vi "FileCreatorMain.vi"() -> ()   [LabVIEW 2017]
uses:
  AutoFileDataType.ctl
panel:
  in  "Flip This Auto":bool
  in  "Auto":T1
  in  "Path File Name":string[](array[string])
  out "standard output":string
  out "standard error":string="NI Linux Real-Time (run mode)\n\nLog in with your NI-Auth credentials.\n\n"
  in  "ExportAllToRobot":bool
  in  "SaveToLocal":bool
  in  "LoadFromLocal":bool
  in  "ExportToRobot":bool
  in  "LoadAllFromRobot":bool
  in  "LocalFiles":i32(listbox)=2
  in  "LocalFileNames":string[](array[string])=["1A.txt", "1B.txt", "1C.txt", "1D.txt", "2A.txt", "2B.txt", "2C.txt", "2D.txt", "3A.txt", "3B.txt", "3C.txt", "3D.txt", "4A.txt", "4B.txt", "4C.txt", "4D.txt"]
  # "Drive:\nWait or\nStart"
  # "Elevator:\nWait or\nStart"
  # "Intake:\nWait or\nStart"
  # "Distance \nfor\nElevator"
  # "Degrees \nto turn"
  # "Elevator\nCommand"
  # "Time for \nintake"
  # "Drive\ncommand"
  # "Time\nfor elevator"
  # "Elevator\n Speed"
  # "Intake \nCommand"
  # "Path File Path"
  # "Speed"
  # "Distance(in)"
  # "Intake Speed"
  # "Drive commands:\n1. For time\n2. For distance\n3. Turn for angle\n4. Stop\n5. Drive Path\n6. Turn To Angle"
  # "Elevator Commands:\n1. For time\n2. To distance\n3. Stop\n4. Pause for time, then distance"
  # "Intake Commands:\n1. For time\n2. Until cube\n3. Stop"
  # "Wait: 0\nStart: 1"
  # "Responses of CMDs run"
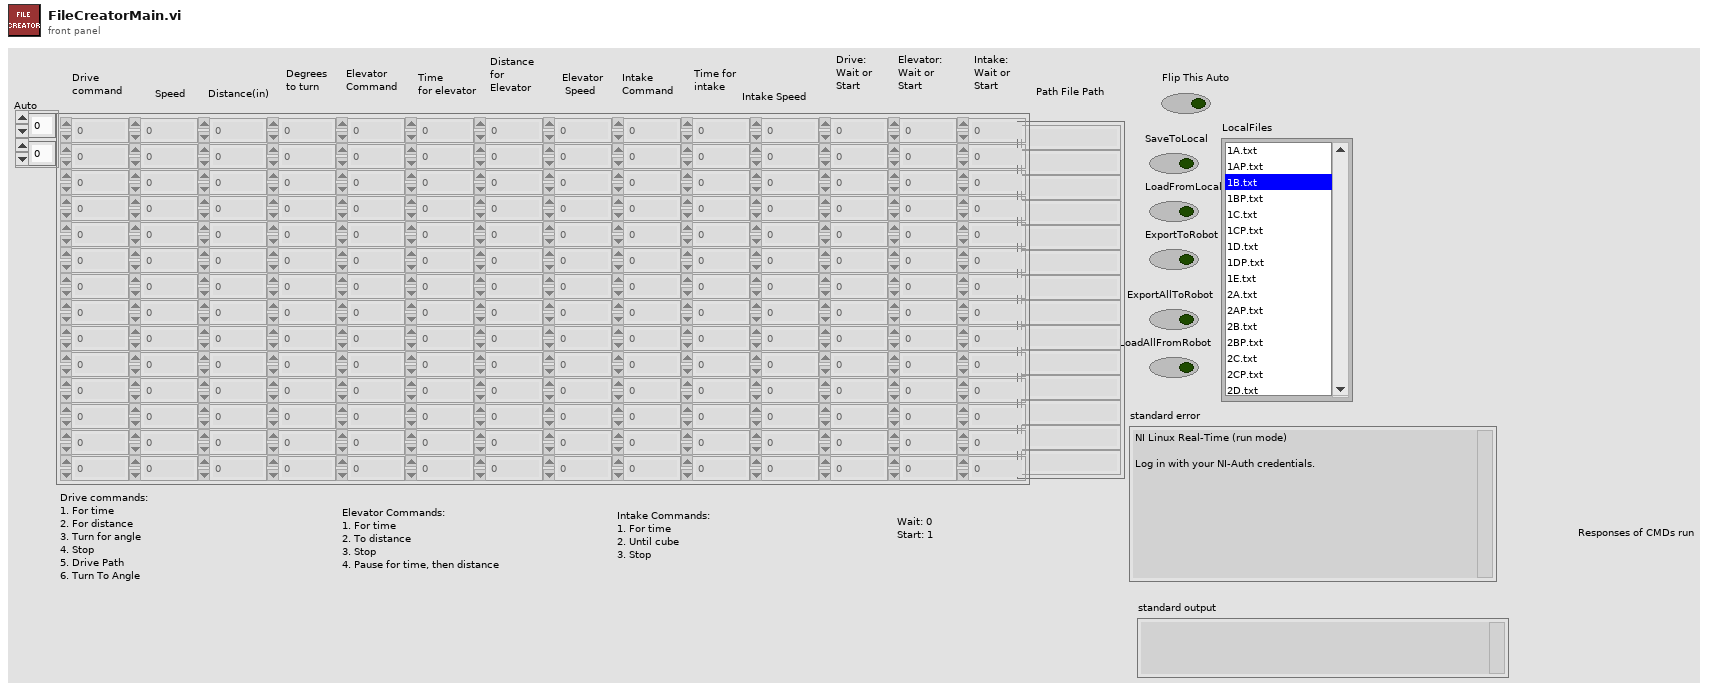
[diagram p1: front panel]
types:
  T1 = typedef "AutoFileDataType.ctl" = dbl[][]
  T2 = enum16{"open", "replace", "create", "open or create", "replace or create", "replace or create with confirmation"}
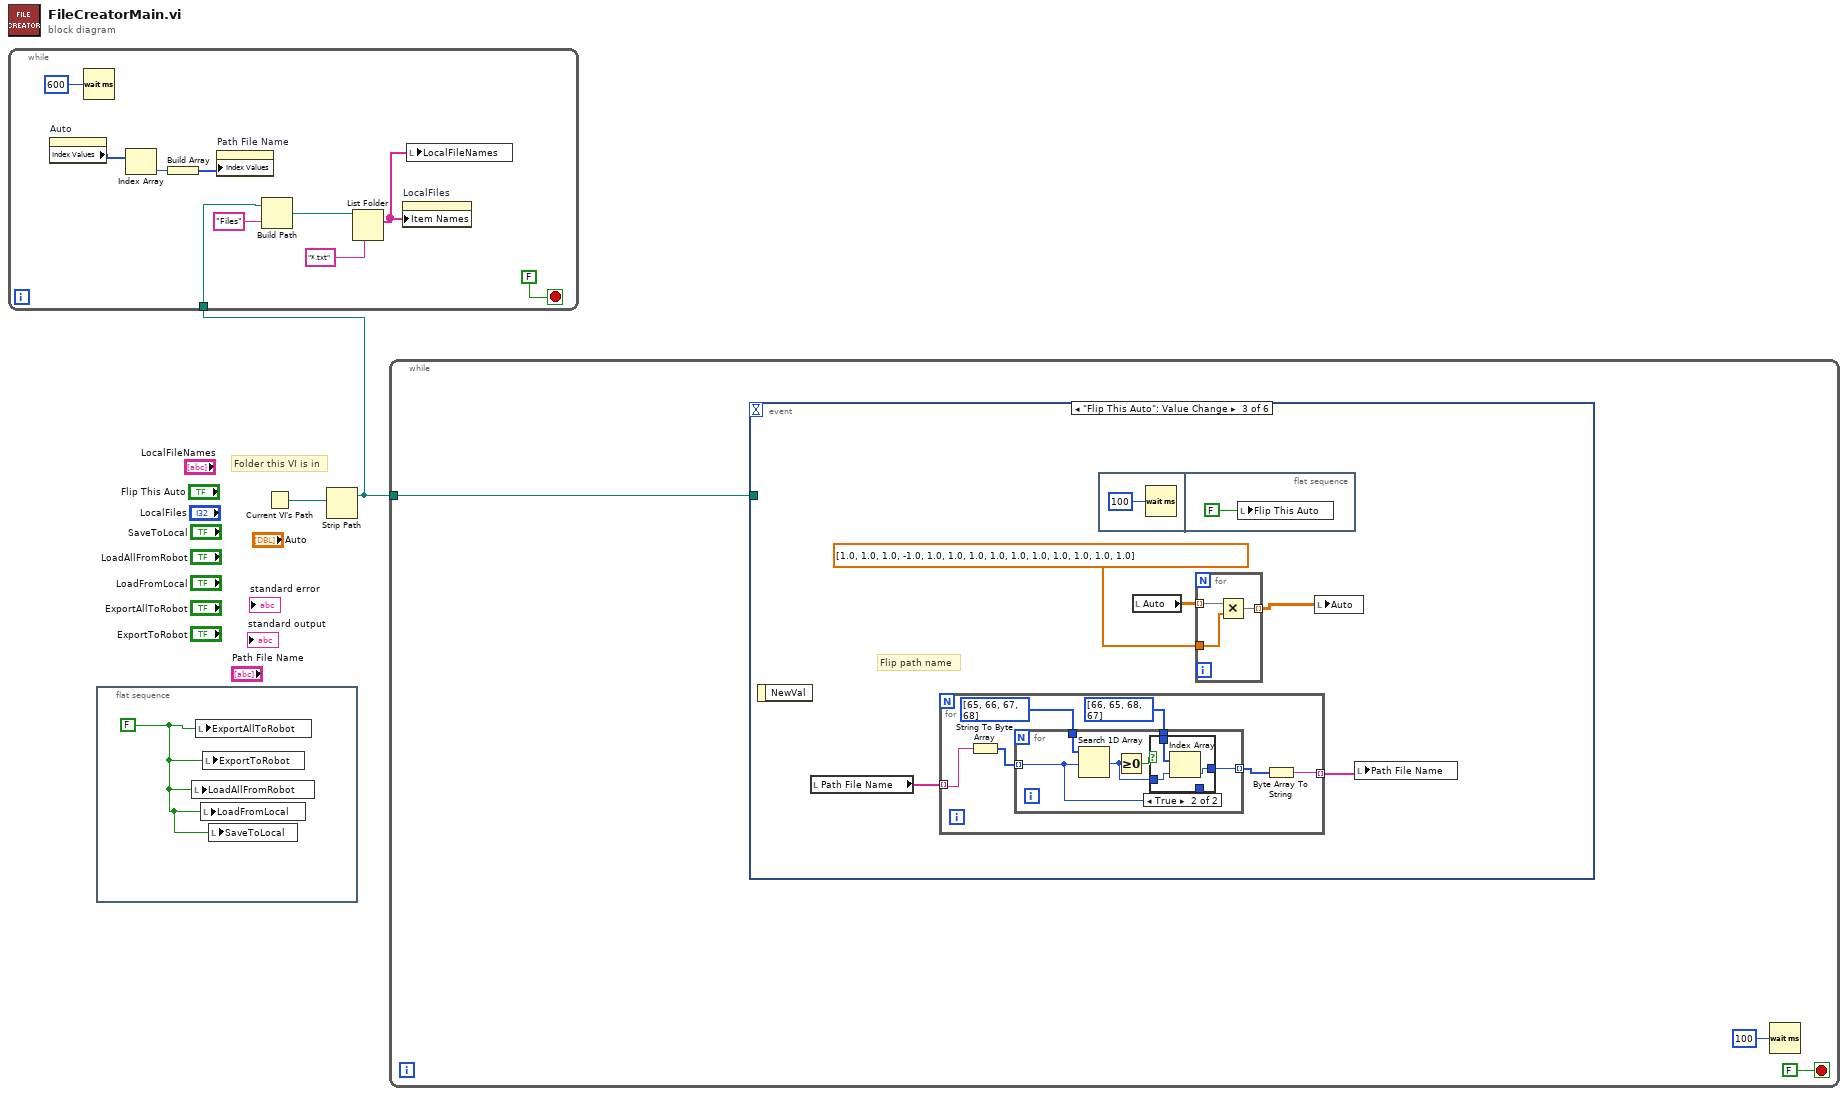
[diagram p0: block diagram]
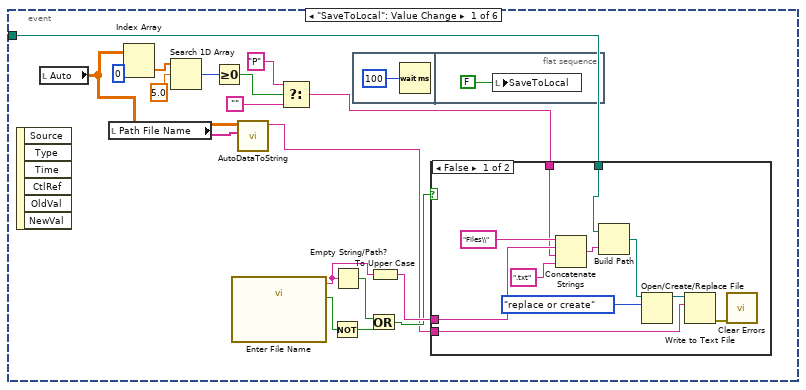
[diagram p2: hidden frame]
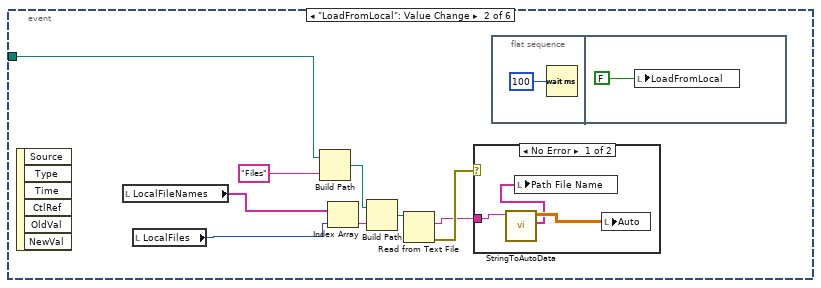
[diagram p4: hidden frame]
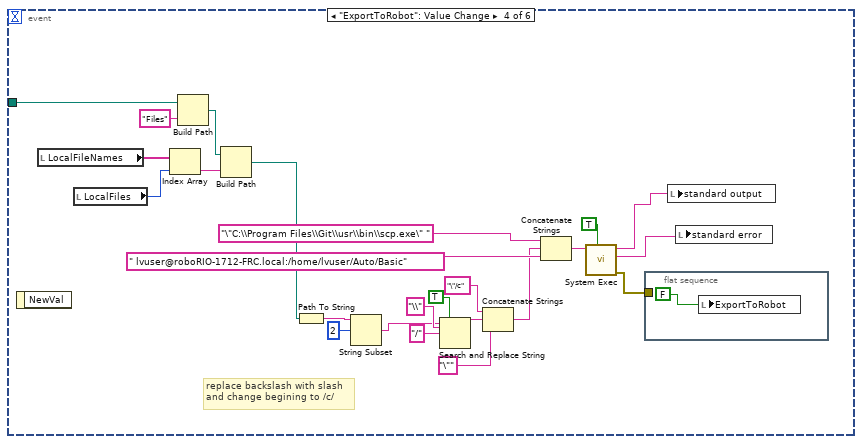
[diagram p7: hidden frame]
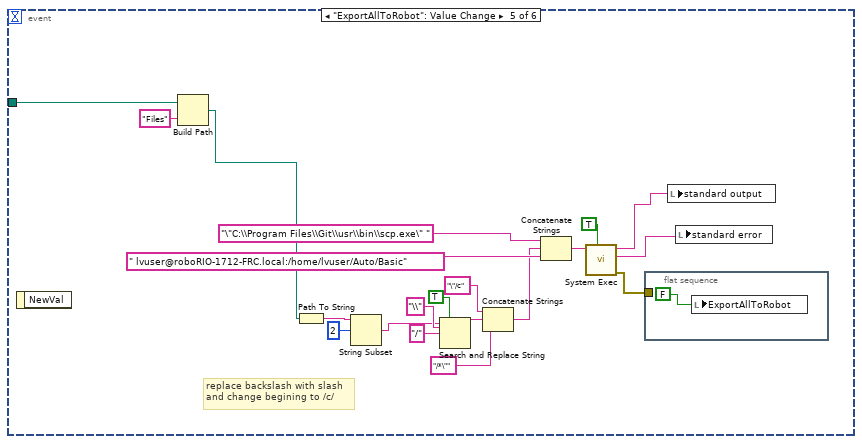
[diagram p8: hidden frame]
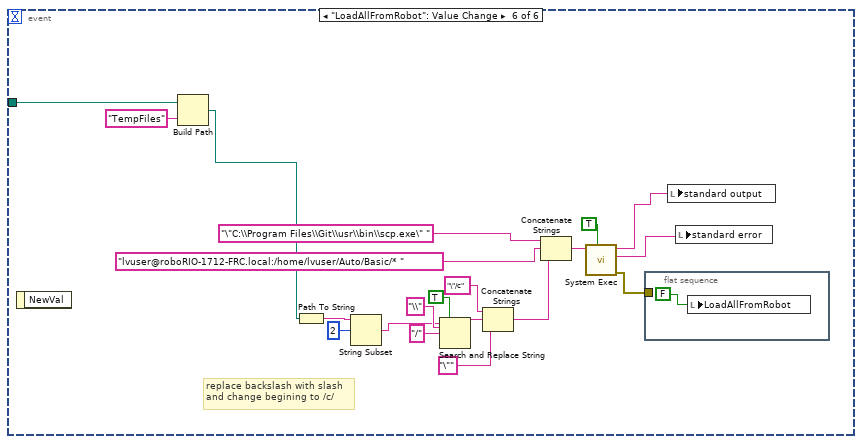
[diagram p9: hidden frame]
diagram:
  # "Folder this VI is in"
  n1 = flat-sequence {
    frame #0 {
      w3 = FALSE ("ExportToRobot")
      n2 = local write "LoadAllFromRobot"(w3) -> ()
      n3 = local write "ExportAllToRobot"(w3) -> ()
      n4 = local write "LoadFromLocal"(w3) -> ()
      n5 = local write "ExportToRobot"(w3) -> ()
      n6 = local write "SaveToLocal"(w3) -> ()
    }
  }
  n7 = Current VI's Path() -> (path=w2:path)
  n8 = Strip Path(path=w2) -> (stripped path=w1:path)  [unwired: 1 out]
  n9 = while {
    tunnel: w1 -> [w9]
    stop <- FALSE stop-if-true
    n10 = property on="Auto" class="Arr (strict)"() -> ("Index Values"=w6:u32[])  [unwired: 2 in, 2 out]
    n11 = Wait (ms)(milliseconds to wait=u32 600) -> ()  [unwired: 1 out]
    n12 = Index Array(array=w6) -> (element=w5:u32)  [unwired: 1 in]
    n13 = Build Array(w5) -> (w4:u32[])
    n14 = property on="Path File Name" class="Arr (strict)"("Index Values"=w4) -> ()  [unwired: 2 in, 2 out]
    n15 = Build Path(base path=w9, name or relative path="Files") -> (appended path=w11:path)
    n16 = List Folder(path=w11, pattern="*.txt") -> (filenames=w7:string[])  [unwired: 2 in, 3 out]
    n17 = property on="LocalFiles" class="LstBox (strict)"("Item Names"=w7) -> ()  [unwired: 2 in, 2 out]
    n18 = local write "LocalFileNames"(w7) -> ()
  }
  n19 = while {
    tunnel: w1 -> [w15]
    stop <- FALSE stop-if-true
    n20 = event shown="[2] \"Flip This Auto\": Value Change" {
      selector: _ -> [_ _ _ _ _ _]
      dyn-events: _ -> [_ _ _ _ _ _]
      timeout: _ -> [_ _ _ _ _ _]
      tunnel: w15 -> [w28 w52 _ w106 w131 w152]
      event "SaveToLocal": Value Change {
        n21 = event-data() -> ()  [unwired: 1 in, 6 out]
        n22 = local read "Auto"() -> (w25:T1)
        n23 = local read "Path File Name"() -> (w26:string[])
        n24 = Index Array(array=w25, index (col)=0 ("disabled index (col)")) -> (element=w24:dbl[])  [unwired: 1 in]
        n25 = Search 1D Array(1D array=w24, element=5.0) -> (index of element=w22:i32)  [unwired: 1 in]
        n26 = Greater Or Equal To 0?(x=w22) -> (x >= 0?=w21:bool)
        n27 = call "Enter File Name"() -> ("File Name"=w31:string, "Enter"=w33:bool)  [unwired: 17 in, 1 out]
        n28 = call "AutoDataToString.vi"("File Path Name"=w26, "Auto"=w25) -> ("String"=w27:string)  [unwired: 9 in]
        n29 = Select(t="P", s=w21, f="") -> (s? t:f=w18:string)
        n30 = Not(x=w33) -> (.not. x?=w32:bool)
        n31 = Empty String/Path?(string/path=w31) -> (empty?=w34:bool)
        n32 = flat-sequence {
          frame #0 {
            n33 = Wait (ms)(milliseconds to wait=u32 100) -> ()  [unwired: 1 out]
          }
          frame #1 {
            n34 = local write "SaveToLocal"(FALSE ("SaveToLocal")) -> ()
          }
        }
        n35 = Or(x=w34, y=w32) -> (x .or. y?=w29:bool)
        n36 = To Upper Case(1:w31) -> (0:w30:string)
        n37 = case shown="False" w29 {
          tunnel: w30 -> [w44 _]
          tunnel: w27 -> [w43 _]
          tunnel: w28 -> [w39 _]
          tunnel: w18 -> [w37 _]
          frame False {
            n38 = Concatenate Strings("Files\\" ("name or relative path"), w44, w37, ".txt" ("string")) -> (w47:string)
            n39 = Build Path(base path=w39, name or relative path=w47) -> (appended path=w42:path)
            n40 = Open/Create/Replace File(file path (use dialog)=w42, operation (0:open)=T2."replace or create") -> (refnum out=w41:refnum<file>)  [unwired: 4 in, 2 out]
            n41 = Write to Text File(file (use dialog)=w41, text=w43) -> (error out=w45:errorcluster)  [unwired: 2 in, 2 out]
            n42 = call <vilib>:"Clear Errors.vi"("error in (no error)"=w45) -> ()  [unwired: 5 in, 2 out]
          }
          frame True {
          }
        }
      }
      event "LoadFromLocal": Value Change {
        n43 = event-data() -> ()  [unwired: 1 in, 6 out]
        n44 = local read "LocalFileNames"() -> (w51:string[])
        n45 = local read "LocalFiles"() -> (w50:i32)
        n46 = Build Path(base path=w52, name or relative path="Files") -> (appended path=w55:path)
        n47 = Index Array(array=w51, index=w50) -> (element=w54:string)
        n48 = Build Path(base path=w55, name or relative path=w54) -> (appended path=w53:path)
        n49 = Read from Text File(file (use dialog)=w53) -> (text=w48:string, error out=w49:errorcluster)  [unwired: 3 in, 2 out]
        n50 = case shown="No Error" w49 {
          tunnel: w48 -> [w61 _]
          frame No Error {
            n51 = call "StringToAutoData.vi"("String"=w61) -> ("Path File Names"=w59:string[], "Auto"=w60:T1)  [unwired: 9 in]
            n52 = local write "Path File Name"(w59) -> ()
            n53 = local write "Auto"(w60) -> ()
          }
          frame Error {
          }
        }
        n54 = flat-sequence {
          frame #0 {
            n55 = Wait (ms)(milliseconds to wait=u32 100) -> ()  [unwired: 1 out]
          }
          frame #1 {
            n56 = local write "LoadFromLocal"(FALSE ("SaveToLocal")) -> ()
          }
        }
      }
      event "Flip This Auto": Value Change {
        # "Flip path name"
        n57 = event-data() -> ()  [unwired: 1 in, 1 out]
        n58 = local read "Path File Name"() -> (w63:string[])
        n59 = for {
          tunnel: w63 -> [w70] mode=indexing
          tunnel: [w68] -> w62 mode=indexing
          n60 = String To Byte Array(string=w70) -> (unsigned byte array=w72:u8[])
          n61 = for {
            tunnel: w72 -> [w75] mode=indexing
            tunnel: u8[] [65, 66, 67, 68] ("1D array") -> [w78]
            tunnel: [w76] -> w69 mode=indexing
            tunnel: u8[] [66, 65, 68, 67] ("1D array") -> [w73]
            n62 = Search 1D Array(1D array=w78, element=w75) -> (index of element=w74:i32)  [unwired: 1 in]
            n63 = Greater Or Equal To 0?(x=w74) -> (x >= 0?=w77:bool)
            n64 = case shown="True" w77 {
              tunnel: [w79 w82] -> w76
              tunnel: w75 -> [w79 _]
              tunnel: w74 -> [_ w81]
              tunnel: w73 -> [_ w80]
              frame False {
              }
              frame True {
                n65 = Index Array(array=w80, index=w81) -> (element=w82:u8)
              }
            }
          }
          n66 = Byte Array To String(unsigned byte array=w69) -> (string=w68:string)
        }
        n67 = flat-sequence {
          frame #0 {
            n68 = Wait (ms)(milliseconds to wait=u32 100) -> ()  [unwired: 1 out]
          }
          frame #1 {
            n69 = local write "Flip This Auto"(FALSE ("Flip This Auto")) -> ()
          }
        }
        n70 = local read "Auto"() -> (w65:T1)
        n71 = for {
          tunnel: dbl[] [1.0, 1.0, 1.0, -1.0, 1.0, 1.0, 1.0, 1.0, 1.0, 1.0, 1.0, 1.0, 1.0, 1.0] -> [w87]
          tunnel: w65 -> [w86] mode=indexing
          tunnel: [w85] -> w64 mode=indexing
          n72 = Multiply(x=w86, y=w87) -> (x*y=w85:dbl[])
        }
        n73 = local write "Auto"(w64) -> ()
        n74 = local write "Path File Name"(w62) -> ()
      }
      event "ExportToRobot": Value Change {
        # "replace backslash with slash\nand change begining to /c/"
        n75 = event-data() -> ()  [unwired: 1 in, 1 out]
        n76 = local read "LocalFileNames"() -> (w109:string[])
        n77 = local read "LocalFiles"() -> (w108:i32)
        n78 = Index Array(array=w109, index=w108) -> (element=w110:string)
        n79 = Build Path(base path=w106, name or relative path="Files") -> (appended path=w111:path)
        n80 = Build Path(base path=w111, name or relative path=w110) -> (appended path=w90:path)
        n81 = Path To String(path=w90) -> (string=w98:string)
        n82 = String Subset(string=w98, offset (0)=2) -> (substring=w96:string)  [unwired: 1 in]
        n83 = Search and Replace String(replace all?=TRUE ("replace all? (F)"), input string=w96, search string="\\", replace string="/" ("replace string (\"\")")) -> (result string=w95:string)  [unwired: 4 in, 3 out]
        n84 = Concatenate Strings("\"/c" ("string"), w95, "\"" ("string")) -> (w93:string)
        n85 = Concatenate Strings("\"C:\\Program Files\\Git\\usr\\bin\\scp.exe\" " ("command line"), w93, " lvuser@roboRIO-1712-FRC.local:/home/lvuser/Auto/Basic" ("string")) -> (w102:string)
        n86 = call <vilib>:"System Exec.vi"("wait until completion? (T)"=TRUE, "command line"=w102) -> ("error out"=w91:errorcluster, "standard error"=w89:string, "standard output"=w88:string)  [unwired: 6 in, 1 out]
        n87 = flat-sequence {
          tunnel: w91 -> [_]
          frame #0 {
            n88 = local write "ExportToRobot"(FALSE ("Export To File")) -> ()
          }
        }
        n89 = local write "standard output"(w88) -> ()
        n90 = local write "standard error"(w89) -> ()
      }
      event "ExportAllToRobot": Value Change {
        # "replace backslash with slash\nand change begining to /c/"
        n91 = event-data() -> ()  [unwired: 1 in, 1 out]
        n92 = Build Path(base path=w131, name or relative path="Files") -> (appended path=w113:path)
        n93 = Path To String(path=w113) -> (string=w123:string)
        n94 = String Subset(string=w123, offset (0)=2) -> (substring=w121:string)  [unwired: 1 in]
        n95 = Search and Replace String(replace all?=TRUE ("replace all? (F)"), input string=w121, search string="\\", replace string="/" ("replace string (\"\")")) -> (result string=w120:string)  [unwired: 4 in, 3 out]
        n96 = Concatenate Strings("\"/c" ("string"), w120, "/*\"" ("string")) -> (w118:string)
        n97 = Concatenate Strings("\"C:\\Program Files\\Git\\usr\\bin\\scp.exe\" " ("command line"), w118, " lvuser@roboRIO-1712-FRC.local:/home/lvuser/Auto/Basic" ("string")) -> (w127:string)
        n98 = call <vilib>:"System Exec.vi"("wait until completion? (T)"=TRUE, "command line"=w127) -> ("error out"=w116:errorcluster, "standard error"=w115:string, "standard output"=w114:string)  [unwired: 6 in, 1 out]
        n99 = flat-sequence {
          tunnel: w116 -> [_]
          frame #0 {
            n100 = local write "ExportAllToRobot"(FALSE ("Export To File")) -> ()
          }
        }
        n101 = local write "standard output"(w114) -> ()
        n102 = local write "standard error"(w115) -> ()
      }
      event "LoadAllFromRobot": Value Change {
        # "replace backslash with slash\nand change begining to /c/"
        n103 = event-data() -> ()  [unwired: 1 in, 1 out]
        n104 = Build Path(base path=w152, name or relative path="TempFiles") -> (appended path=w136:path)
        n105 = Path To String(path=w136) -> (string=w145:string)
        n106 = String Subset(string=w145, offset (0)=2) -> (substring=w143:string)  [unwired: 1 in]
        n107 = Search and Replace String(replace all?=TRUE ("replace all? (F)"), input string=w143, search string="\\", replace string="/" ("replace string (\"\")")) -> (result string=w142:string)  [unwired: 4 in, 3 out]
        n108 = Concatenate Strings("\"/c" ("string"), w142, "\"" ("string")) -> (w134:string)
        n109 = Concatenate Strings("\"C:\\Program Files\\Git\\usr\\bin\\scp.exe\" " ("command line"), "lvuser@roboRIO-1712-FRC.local:/home/lvuser/Auto/Basic/* " ("string"), w134) -> (w149:string)
        n110 = call <vilib>:"System Exec.vi"("wait until completion? (T)"=TRUE, "command line"=w149) -> ("error out"=w139:errorcluster, "standard error"=w138:string, "standard output"=w137:string)  [unwired: 6 in, 1 out]
        n111 = flat-sequence {
          tunnel: w139 -> [_]
          frame #0 {
            n112 = local write "LoadAllFromRobot"(FALSE ("Export To File")) -> ()
          }
        }
        n113 = local write "standard output"(w137) -> ()
        n114 = local write "standard error"(w138) -> ()
      }
    }
    n115 = Wait (ms)(milliseconds to wait=u32 100) -> ()  [unwired: 1 out]
  }
